vi "test default class value.vi"() -> ()   [LabVIEW 2012]
panel:
  out "error out":errorcluster
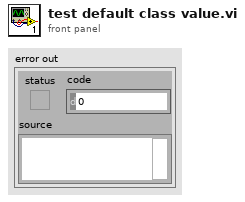
[diagram p1: front panel]
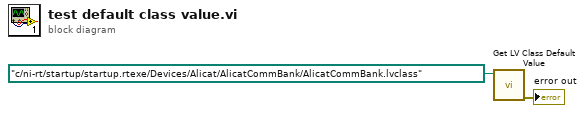
[diagram p0: block diagram]
diagram:
  n1 = call <vilib>:"Get LV Class Default Value.vi"("class path"=path "c:/ni-rt/startup/startup.rtexe/Devices/Alicat/AlicatCommBank/AlicatCommBank.lvclass") -> ("error out"=→"error out":errorcluster)  [unwired: 9 in, 1 out]
